vi "Uninstall Package.vi"(8 "error in":errorcluster, 11 "package name":string) -> (0 "error out":errorcluster, 3 "package name out":string)   [LabVIEW 2014, in "NIPM_API.lvlib"]
doc: "Uninstalls the specified package on this computer.\n\nNOTE: This VI does not work when the package installation requires admin priviledges (e.g. package installs files to Program Files directory)."
uses:
  NIPM_API.lvlib
panel:
  out "command line standard output":string
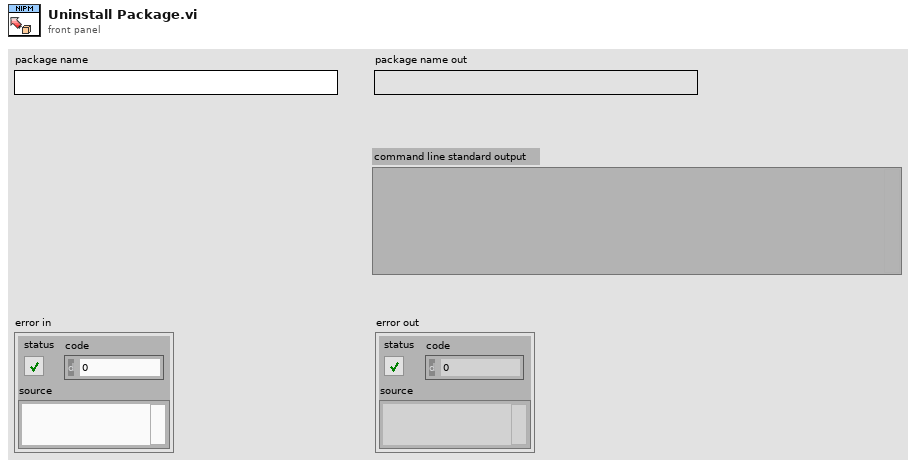
[diagram p1: front panel]
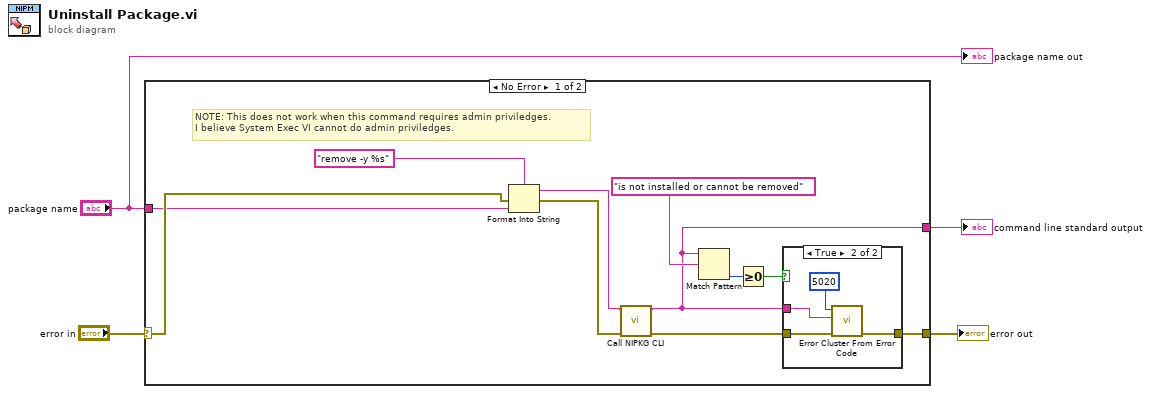
[diagram p0: block diagram]
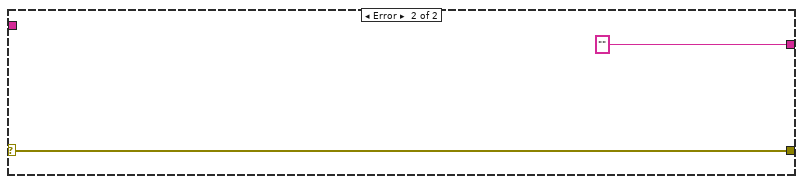
[diagram p3: hidden frame]
diagram:
  n1 = case shown="No Error" "error in" {
    selector: "error in" -> [w14 w22]
    tunnel: [w7 w22] -> w3
    tunnel: [w6 "" ("command line standard output")] -> w2
    tunnel: "package name" -> [w5 _]
    frame No Error {
      # "NOTE: This does not work when this command requires admin priviledges.\nI believe System Exec VI cannot do admin priviledges."
      n2 = Format Into String(format string="remove -y %s", error in=w14, w5) -> (resulting string=w12:string, error out=w13:errorcluster)  [unwired: 1 in]
      n3 = call "Call NIPKG CLI.vi"("error in (no error)"=w13, "command"=w12) -> ("error out"=w8:errorcluster, "command line standard output"=w6:string)  [unwired: 8 in]
      n4 = Match Pattern(string=w6, regular expression="is not installed or cannot be removed") -> (offset past match=w10:i32)  [unwired: 1 in, 3 out]
      n5 = Greater Or Equal To 0?(x=w10) -> (x >= 0?=w9:bool)
      n6 = case shown="True" w9 {
        tunnel: w8 -> [w16 w19]
        tunnel: [w16 w18] -> w7
        tunnel: w6 -> [_ w17]
        frame False {
        }
        frame True {
          n7 = call <vilib>:"Error Cluster From Error Code.vi"("error in (no error)"=w19, "error message (\"\")"=w17, "error code (0)"=5020) -> ("error out"=w18:errorcluster)  [unwired: 6 in]
        }
      }
    }
    frame Error {
    }
  }
  "error out" <- w3
  "command line standard output" <- w2
  "package name out" <- "package name"
